vi "Clear Annotations.vi"(8 "error in (no error)":errorcluster, 11 "FSM in":refnum<class "FSM.Graph.lvclass">) -> (0 "error out":errorcluster, 3 "FSM out":refnum<class "FSM.Graph.lvclass">)   [LabVIEW 2015, in "FSM.Graph.lvclass"]
uses:
  FSM.Graph.lvclass
  FSM.Graph.lvclass/FSM.Graph.ctl
  FSM.Edge/FSM.Edge.lvclass
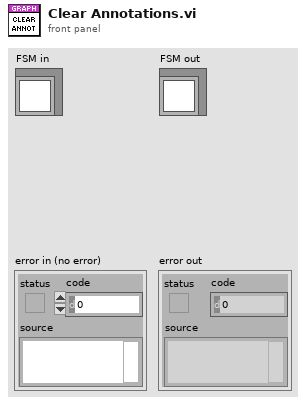
[diagram p1: front panel]
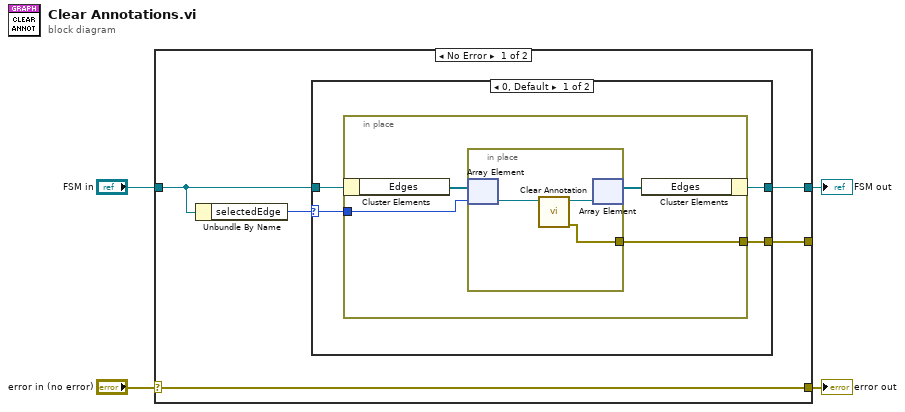
[diagram p0: block diagram]
diagram:
  n1 = case shown="No Error" "error in (no error)" {
    selector: "error in (no error)" -> [w9 w23]
    tunnel: [w9 w23] -> w3
    tunnel: [w6 w22] -> w1
    tunnel: "FSM in" -> [w7 w22]
    tunnel: [w5 _] -> _
    frame No Error {
      n2 = Unbundle By Name(w7) -> ("selectedEdge"=w8:i32)
      n3 = case shown="0, Default" w8 {
        selector: w8 -> [w12 _]
        tunnel: w7 -> [w13 w21]
        tunnel: [w11 w21] -> w6
        tunnel: [w10 _] -> w5
        frame 0, Default {
          n4 = in-place {
            in-place-border: w12 -> [w16]
            in-place-border: [w14] -> w10
            n5 = in-place-cluster #1(w13) -> ("Edges"=w17:refnum<class "FSM.Edge.lvclass">[])
            n6 = in-place {
              in-place-border: [w18] -> w14
              n7 = in-place-array #2(w17, w16) -> (w20:refnum<class "FSM.Edge.lvclass">)
              n8 = call "Clear Annotation.vi"("FSM.Edge in"=w20) -> ("error out"=w18:errorcluster, "FSM.Edge out"=w19:refnum<class "FSM.Edge.lvclass">)  [unwired: 9 in]
              n9 = in-place-array #2(w19) -> (w15:refnum<class "FSM.Edge.lvclass">[])  [unwired: 1 out]
            }
            n10 = in-place-cluster #1("Edges"=w15) -> (w11:refnum<class "FSM.Graph.lvclass">)
          }
        }
        frame -1 {
        }
      }
    }
    frame Error {
    }
  }
  "error out" <- w3
  "FSM out" <- w1
